vi "Tamer GV.vi"() -> ()   [LabVIEW 2020, in "Tamer.lvlib" / "Tamer.lvclass"]
uses:
  Tamer.lvclass
  Tamer Status.ctl
  Monkey Summary.ctl
  Run Utilities/TypeDefs/Monkey Status.ctl
  Link Chain GUI.ctl
  Run Utilities/Run Utilities.lvlib
panel:
  out "Tamer Panel":T1
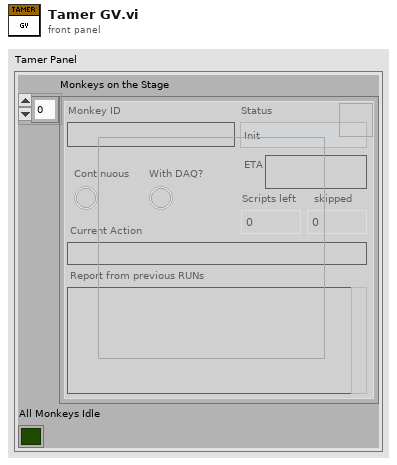
[diagram p1: front panel]
types:
  T1 = typedef "Tamer.lvlib/Tamer.lvclass/Tamer Status.ctl" = cluster{"Monkeys on the Stage":T2[], "All Monkeys Idle":bool}
  T2 = typedef "Tamer.lvlib/Tamer.lvclass/Monkey Summary.ctl" = cluster{"Color":u32, "Status":T3, "Continuous":bool, "Scripts left":u32, "Scripts skipped":u32, "ETA":string, "Current Action":string, "Report from previous RUNs":string, "Monkey ID":string, "With DAQ?":bool, "Linked?":T4, "Paused":bool}
  T3 = typedef "TALOS.lvlib/Run Utilities.lvlib/Monkey Status.ctl" = enum16{"Init", "Paused", "Ongoing", "Stopped", "Finished (no errors)", "Finished (with errors)"}
  T4 = typedef "Tamer.lvlib/Tamer.lvclass/Link Chain GUI.ctl" = bool
diagram:
